vi "Set SRX PID.vi"(7 "subsystem":string, 9 "Setpoint":dbl, 11 "CAN Talon SRX Ref":T1={"DeviceStatus"={"status"=FALSE, "code"=0, "source"=""}, "Type"=enum."PWM", "PWM"={"PWM Channel"=enum."PWM 1", "DeadBand"={"Name"="", "maxPositivePwm"=0, "minPositivePwm"=0, "centerPwm"=0, "maxNegativePwm"=0, "minNegativePwm"=0, "angularRange"=0}}, "CAN"={"Device Number"=0, "Control Mode"=enum."Percent VBus", "Semaphore"=refnum, "Max Vout"=12.0, "TalonSRX Control Mode"=enum."Percent VBus"}, "Invert"=FALSE}) -> (3 "MotorControlDevRef":T1={"DeviceStatus"={"status"=FALSE, "code"=0, "source"=""}, "Type"=enum."PWM", "PWM"={"PWM Channel"=enum."Invalid", "DeadBand"={"Name"="", "maxPositivePwm"=0, "minPositivePwm"=0, "centerPwm"=0, "maxNegativePwm"=0, "minNegativePwm"=0, "angularRange"=0}}, "CAN"={"Device Number"=0, "Control Mode"=enum."Percent VBus", "Semaphore"=refnum, "Max Vout"=12.0, "TalonSRX Control Mode"=enum."Percent VBus"}, "Invert"=FALSE})   [LabVIEW 2015]
uses:
  <vilib>/Rock Robotics/WPI/MotorControl/WPI_MotorControlDeviceRef.ctl
  <vilib>/Rock Robotics/WPI/MotorControl/WPI_MotorControlType.ctl
  <vilib>/Rock Robotics/SystemInterfaces/DIO/FPGA_DIOPWMChannel.ctl
  <vilib>/Rock Robotics/WPI/PWM/WPI_PWMDeadband.ctl
  <vilib>/Rock Robotics/WPI/CAN/Jaguar/SubVIs/WPI_CANJaguar_ControlMode.ctl
  <vilib>/Rock Robotics/WPI/CAN/TalonSRX/WPI_CANTalonSRX_APIControlMode.ctl
  <vilib>/Rock Robotics/Network Tables/NT Read Number.vi
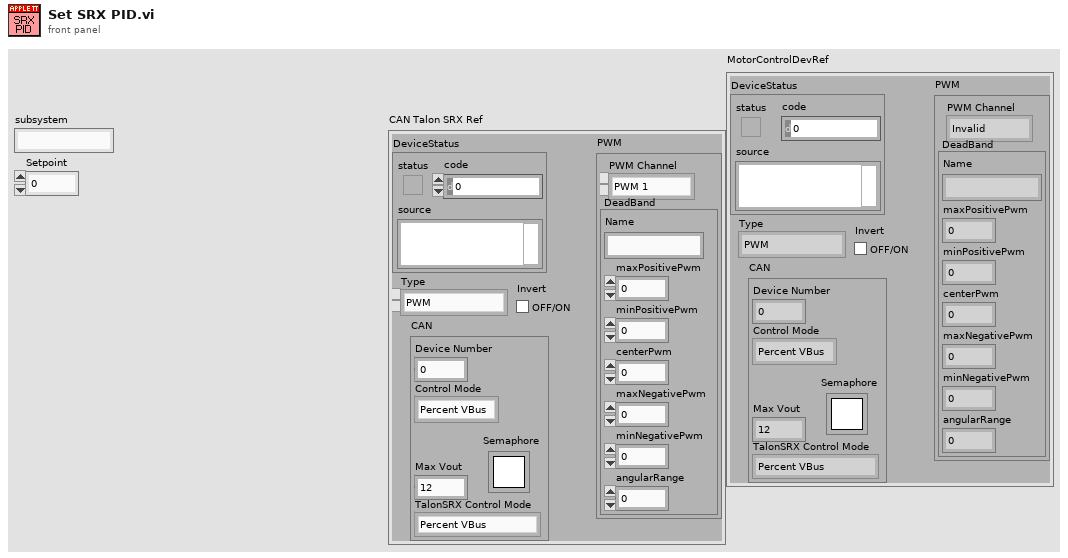
[diagram p1: front panel]
types:
  T1 = typedef "WPI_MotorControlDeviceRef.ctl" = cluster{"DeviceStatus":errorcluster, "Type":T2, "PWM":cluster{"PWM Channel":T3, "DeadBand":T4}, "CAN":cluster{"Device Number":u8, "Control Mode":T5, "Semaphore":T6, "Max Vout":dbl, "TalonSRX Control Mode":T7}, "Invert":bool}
  T2 = typedef "WPI_MotorControlType.ctl" = enum16{"PWM", "CAN", "CANTalonSRX"}
  T3 = typedef "FPGA_DIOPWMChannel.ctl" = enum8{"PWM 0", "PWM 1", "PWM 2", "PWM 3", "PWM 4", "PWM 5", "PWM 6", "PWM 7", "PWM 8", "PWM 9", "PWM MXP 0", "PWM MXP 1", "PWM MXP 2", "PWM MXP 3", "PWM MXP 4", "PWM MXP 5", "PWM MXP 6", "PWM MXP 7", "PWM MXP 8", "PWM MXP 9", "Invalid"}
  T4 = typedef "WPI_PWMDeadband.ctl" = cluster{"Name":string, "maxPositivePwm":i32, "minPositivePwm":i32, "centerPwm":i32, "maxNegativePwm":i32, "minNegativePwm":i32, "angularRange":u16}
  T5 = typedef "WPI_CANJaguar_ControlMode.ctl" = enum8{"Percent VBus", "Current", "Speed", "Position", "Voltage"}
  T6 = typedef "Semaphore RefNum" = refnum<k1>
  T7 = typedef "WPI_CANTalonSRX_APIControlMode.ctl" = enum8{"Percent VBus", "Speed", "Position", "Slave", "Unchanged / Invalid", "Voltage Compensation", "Current", "Motion Profile"}
  T8 = cluster{"proportional gain (Kc)":dbl, "integral time (Ti, min)":dbl, "derivative time (Td, min)":dbl}
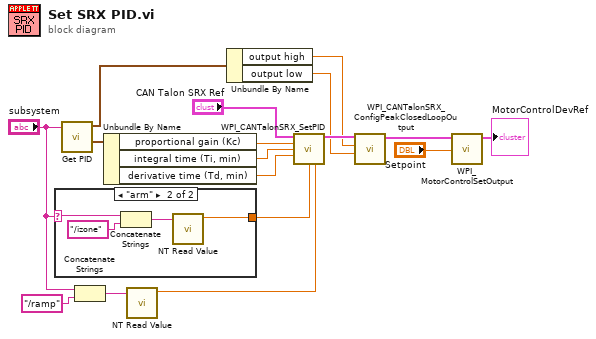
[diagram p0: block diagram]
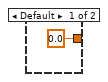
[diagram p2: hidden frame]
diagram:
  n1 = case shown="\"arm\"" "subsystem" {
    selector: "subsystem" -> [_ w20]
    tunnel: [0.0 ("Numeric") w19] -> w7
    frame Default {
    }
    frame "arm" {
      n2 = Concatenate Strings(w20, "/izone") -> (w21:string)
      n3 = call-poly <vilib>:"NT Read Value.vi"("Name"=w21) -> ("Numeric"=w19:dbl)  [unwired: 9 in, 1 out]
    }
  }
  n4 = call "Get PID.vi"("Subsystem"="subsystem") -> ("PID Gains"=w16:T8, "output range"=w6:cluster{"output high":dbl, "output low":dbl})  [unwired: 8 in]
  n5 = Concatenate Strings("subsystem", "/ramp") -> (w10:string)
  n6 = Unbundle By Name(w16) -> ("proportional gain (Kc)"=w15:dbl, "integral time (Ti, min)"=w13:dbl, "derivative time (Td, min)"=w12:dbl)
  n7 = call-poly <vilib>:"NT Read Value.vi"("Name"=w10) -> ("Numeric"=w9:dbl)  [unwired: 9 in, 1 out]
  n8 = Unbundle By Name(w6) -> ("output high"=w4:dbl, "output low"=w5:dbl)
  n9 = call <vilib>:"WPI_CANTalonSRX_SetPID.vi"("CAN Talon SRX Ref"="CAN Talon SRX Ref", "P"=w15, "I"=w13, "D"=w12, "I Zone"=w7, "Ramp Rate"=w9) -> ("CAN Talon SRX Ref"=w17:T1)  [unwired: 8 in, 1 out]
  n10 = call <vilib>:"WPI_CANTalonSRX_ConfigPeakClosedLoopOutput.vi"("Reverse Peak Output"=w5, "Forward Peak Output"=w4, "CAN Talon SRX Ref"=w17) -> ("CAN Talon SRX Ref"=w3:T1)  [unwired: 7 in, 1 out]
  n11 = call <vilib>:"WPI_MotorControlSetOutput.vi"("Output"="Setpoint", "MotorControlDevRef"=w3) -> ("MotorControlDevRef"=→"MotorControlDevRef":T1)  [unwired: 7 in, 2 out]
